vi "ReadFile.vi"(8 "error in (no error)":errorcluster, 11 "RWFile in":refnum<class "RWFile.lvclass">) -> (0 "error out":errorcluster, 2 "data":i32[](array[numeric]))   [LabVIEW 2021, in "RWFile.lvclass"]
uses:
  RWFile.lvclass
  RWFile.lvclass/RWFile.ctl
  File/File.lvclass
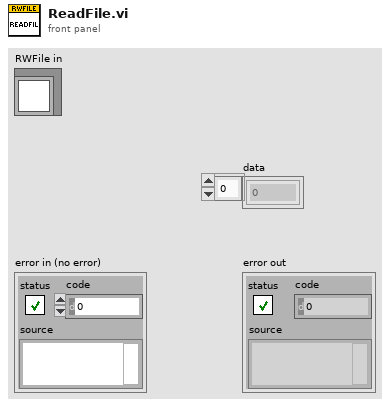
[diagram p1: front panel]
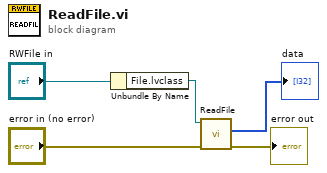
[diagram p0: block diagram]
diagram:
  n1 = Unbundle By Name("RWFile in") -> ("File.lvclass"=w2:refnum<class "File.lvclass">)
  n2 = call "ReadFile.vi"("error in (no error)"="error in (no error)", "File in"=w2) -> ("error out"=→"error out":errorcluster, "data"=→"data":i32[])  [unwired: 8 in]
